vi "Simple Add3.vi"() -> ()   [LabVIEW 2016]
panel:
  out "Answer":dbl
  in  "Y":dbl
  in  "X":dbl
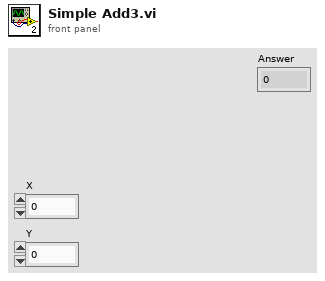
[diagram p1: front panel]
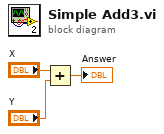
[diagram p0: block diagram]
diagram:
  n1 = Add(x="X", y="Y") -> (x+y=→"Answer":dbl)
